vi "Controller Acquisition and Actuation Loop.vi"(4 "Iteration duration":u64, 5 "Missed iteration count":u32, 6 "Timestamp":u64, 7 "Sync Objects":T3, 8 "error in (no error)":errorcluster, 9 "PS Variables":T1, 10 "BPM Variables":T2, 11 "FOFB Configuration":T6={"FOFB Parameters"={"Network"={"FOFB Controller IP"="", "LNLS Control Network IP"="", "LNLS Control Network Power Supplies TCP Port"=0, "LNLS Control Network FOFB Configuration TCP Port"=0, "LNLS Control Network BPMs TCP Port"=0, "Monitoring Data TCP Port"=0, "Fast Archiver TCP Port"=0, "Fast Command TCP Port"=0, "TCP Listening Timeout"=0}, "Fast Acquisition"={"Sampling Period"=0, "Data Buffer Size"=0, "Monitoring Period"=0}, "Acquisition Network"=[], "Actuation Network"=[]}, "Number of Acquisition Chassis"=0, "Number of Actuation Chassis"=0, "Number of BPM Readings"=0, "BPM Reading Names"=[], "Selected BPM Readings"=[0, 1, 2, 3, 4, 5, 6, 7, 8, 9, 10, 11, 12, 13, 14, 15, 16, 17, 18, 19, 20, 21, 22, 23, 24, 25, 26, 27, 28, 29, 30, 31, 32, 33, 34, 35, 36, 37, 38, 39, 40, 41, 42, 43, 44, 45, 46, 47, 48, 49], "Number of Correctors"=0, "Corrector Names"=[], "Selected Correctors"=[0, 1, 2, 3, 4, 5, 6, 7, 8, 9, 10, 11, 12, 13, 14, 15, 16, 17, 18, 19, 20, 21, 22, 23, 24, 25, 26, 27, 28, 29, 30, 31, 32, 33, 34, 35, 36, 37, 38, 39, 40, 41, 42, 43, 44, 45, 46, 47, 48, 49], "Response Matrix"=[], "Reference Orbit"=[], "Correction Matrix"=[], "FPGA Filter Sets"=[], "Acquisition Chassis Names"=[], "Actuation Chassis Names"=[], "Acquisition Variables"=[], "Actuation Variables"=[], "PS Matrix Mapping"=[], "Inverse PS Matrix Mapping"=[], "BPM Matrix Mapping"=[], "Inverse BPM Matrix Mapping"=[], "BPM Planes"=[], "Corrector Planes"=[]}) -> (0 "error out":errorcluster)   [LabVIEW 2011, in "Controller VIs.lvlib"]
doc: "Continuously performs acquisition of all input variables (BPM readings, Power Supply readings, etc.) and forwards data to the <b>Decimated Acquisition Loop</b>."
uses:
  Controller VIs.lvlib
  Types Definitions/Type FOFB Configuration.ctl
  Types Definitions/Type FOFB Parameters.ctl
  Types Definitions/Type Network Configuration.ctl
  Types Definitions/Type FA Configuration.ctl
  Types Definitions/Type Acquisition Network Configuration.ctl
  Types Definitions/Type Actuation Network Configuration.ctl
  Types Definitions/Type Synchronization Objects.ctl
  Types Definitions/Type Blocking Synchronization Objects.ctl
  Types Definitions/Type Monitoring Data.ctl
  Types Definitions/Type Operation Mode State.ctl
  Types Definitions/Type Diagnostics Data.ctl
  Types Definitions/Type CPU Loads Array.ctl
  Types Definitions/Type CPU Loads.ctl
  Types Definitions/Type Non-blocking Synchronization Objects.ctl
  Types Definitions/Type FOFB Variables.ctl
  Types Definitions/Type Actuation State.ctl
  Types Definitions/Type BPM Variables.ctl
  Types Definitions/Type PS Variables.ctl
  Controller Write UINT8.vi
  Controller Write PS Setpoints.vi
  Controller Write Boolean.vi
  Controller Write FXP22.4.vi
  Controller Write UINT16.vi
  Controller Read FXP20.5.vi
  Controller Read UINT8.vi
  Controller Write FXP20.5.vi
  Type Definitions.lvlib
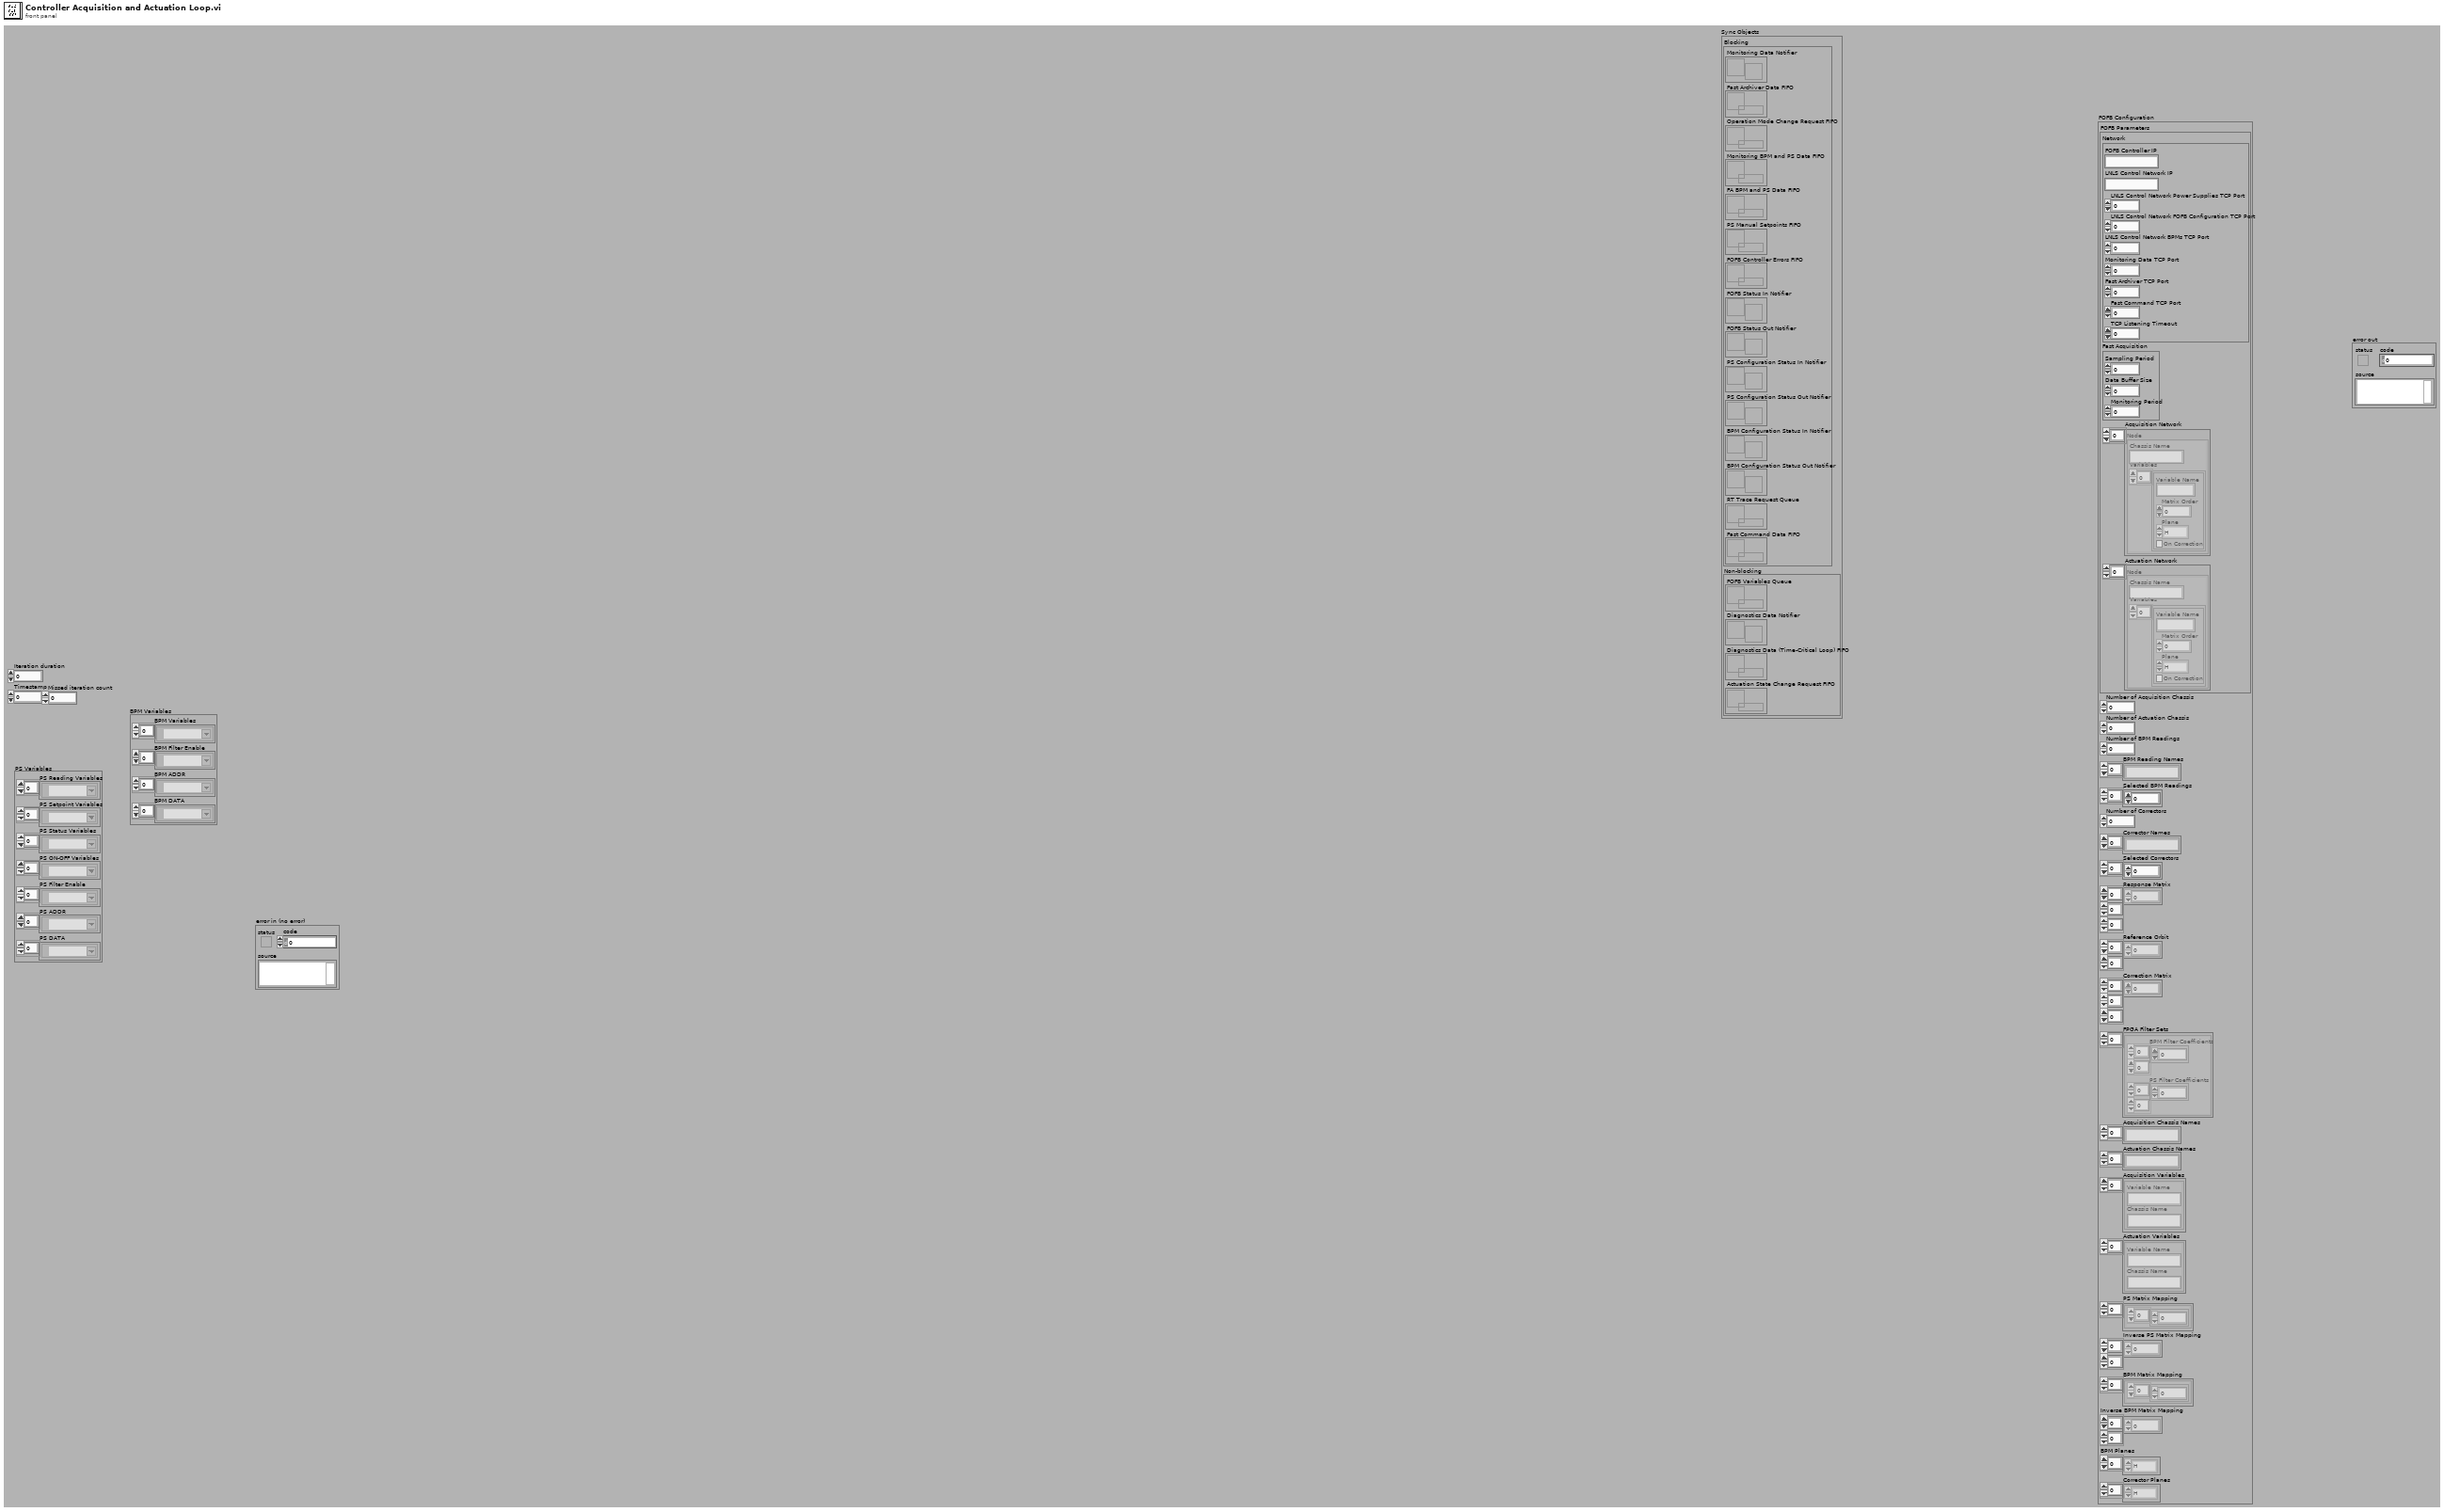
[diagram p1: front panel]
types:
  T1 = typedef "Type Definitions.lvlib/Type PS Variables.ctl" = cluster{"PS Reading Variables":refnum<k21>[], "PS Setpoint Variables":refnum<k21>[], "PS Status Variables":refnum<k21>[], "PS ON-OFF Variables":refnum<k21>[], "PS Filter Enable":refnum<k21>[], "PS ADDR":refnum<k21>[], "PS DATA":refnum<k21>[]}
  T2 = typedef "Type Definitions.lvlib/Type BPM Variables.ctl" = cluster{"BPM Variables":refnum<k21>[], "BPM Filter Enable":refnum<k21>[], "BPM ADDR":refnum<k21>[], "BPM DATA":refnum<k21>[]}
  T3 = typedef "Type Definitions.lvlib/Type Synchronization Objects.ctl" = cluster{"Blocking":T4, "Non-blocking":T5}
  T4 = typedef "Type Definitions.lvlib/Type Blocking Synchronization Objects.ctl" = cluster{"Monitoring Data Notifier":refnum<notifier>, "Fast Archiver Data FIFO":refnum<queue>, "Operation Mode Change Request FIFO":refnum<k33>, "Monitoring BPM and PS Data FIFO":refnum<k33>, "FA BPM and PS Data FIFO":refnum<k33>, "PS Manual Setpoints FIFO":refnum<k33>, "FOFB Controller Errors FIFO ":refnum<k33>, "FOFB Status In Notifier":refnum<notifier>, "FOFB Status Out Notifier":refnum<notifier>, "PS Configuration Status In Notifier":refnum<notifier>, "PS Configuration Status Out Notifier":refnum<notifier>, "BPM Configuration Status In Notifier":refnum<notifier>, "BPM Configuration Status Out Notifier":refnum<notifier>, "RT Trace Request Queue":refnum<queue>, "Fast Command Data FIFO":refnum<k33>}
  T5 = typedef "Type Definitions.lvlib/Type Non-blocking Synchronization Objects.ctl" = cluster{"FOFB Variables Queue":refnum<queue>, "Diagnostics Data Notifier":refnum<notifier>, "Diagnostics Data (Time-Critical Loop) FIFO":refnum<k33>, "Actuation State Change Request FIFO":refnum<k33>}
  T6 = typedef "Type Definitions.lvlib/Type FOFB Configuration.ctl" = cluster{"FOFB Parameters":T7, "Number of Acquisition Chassis":i32, "Number of Actuation Chassis":i32, "Number of BPM Readings":i32, "BPM Reading Names":string[], "Selected BPM Readings":u32[], "Number of Correctors":i32, "Corrector Names":string[], "Selected Correctors":u32[], "Response Matrix":dbl[][][], "Reference Orbit":dbl[][], "Correction Matrix":dbl[][][], "FPGA Filter Sets":cluster{"BPM Filter Coefficients":dbl[][], "PS Filter Coefficients":dbl[][]}[], "Acquisition Chassis Names":string[], "Actuation Chassis Names":string[], "Acquisition Variables":cluster{"Variable Name":string, "Chassis Name":string}[], "Actuation Variables":cluster{"Variable Name":string, "Chassis Name":string}[], "PS Matrix Mapping":cluster{u32[]}[], "Inverse PS Matrix Mapping":u32[][], "BPM Matrix Mapping":cluster{u32[]}[], "Inverse BPM Matrix Mapping":u32[][], "BPM Planes":enum8{"H", "V"}[], "Corrector Planes":enum8{"H", "V"}[]}
  T7 = typedef "Type Definitions.lvlib/Type FOFB Parameters.ctl" = cluster{"Network":T8, "Fast Acquisition":T9, "Acquisition Network":T10, "Actuation Network":T11}
  T8 = typedef "Type Definitions.lvlib/Type Network Configuration.ctl" = cluster{"FOFB Controller IP":string, "LNLS Control Network IP":string, "LNLS Control Network Power Supplies TCP Port":u16, "LNLS Control Network FOFB Configuration TCP Port":u16, "LNLS Control Network BPMs TCP Port":u16, "Monitoring Data TCP Port":u16, "Fast Archiver TCP Port":u16, "Fast Command TCP Port":u16, "TCP Listening Timeout":i32}
  T9 = typedef "Type Definitions.lvlib/Type FA Configuration.ctl" = cluster{"Sampling Period":u32, "Data Buffer Size":u32, "Monitoring Period":u32}
  T10 = typedef "Type Definitions.lvlib/Type Acquisition Network Configuration.ctl" = cluster{"Chassis Name":string, "Variables":cluster{"Variable Name":string, "Matrix Order":u32, "Plane":enum8{"H", "V"}, "On Correction":bool}[]}[]
  T11 = typedef "Type Definitions.lvlib/Type Actuation Network Configuration.ctl" = cluster{"Chassis Name":string, "Variables":cluster{"Variable Name":string, "Matrix Order":u32, "Plane":enum8{"H", "V"}, "On Correction":bool}[]}[]
  T12 = typedef "Type Definitions.lvlib/Type Actuation State.ctl" = enum8{"Only reading", "Manual", "FOFB Initialization", "FOFB", "FOFB Stopping"}
  T13 = typedef "Type Definitions.lvlib/Type FOFB Variables.ctl" = cluster{"Reference Orbit":dbl[], "Response Matrix":dbl[][], "Correction Matrix":dbl[][], "FPGA Filter":cluster{"BPM Filter Coefficients":dbl[][], "PS Filter Coefficients":dbl[][]}, "Selected BPM Readings":u32[], "Selected Correctors":u32[], "BPM Planes":enum8{"H", "V"}[], "Corrector Planes":enum8{"H", "V"}[], "Fast Command Enabled":bool, "Horizontal Gain":dbl, "Vertical Gain":dbl, "Horizontal Distortion Threshold":dbl, "Vertical Distortion Threshold":dbl}
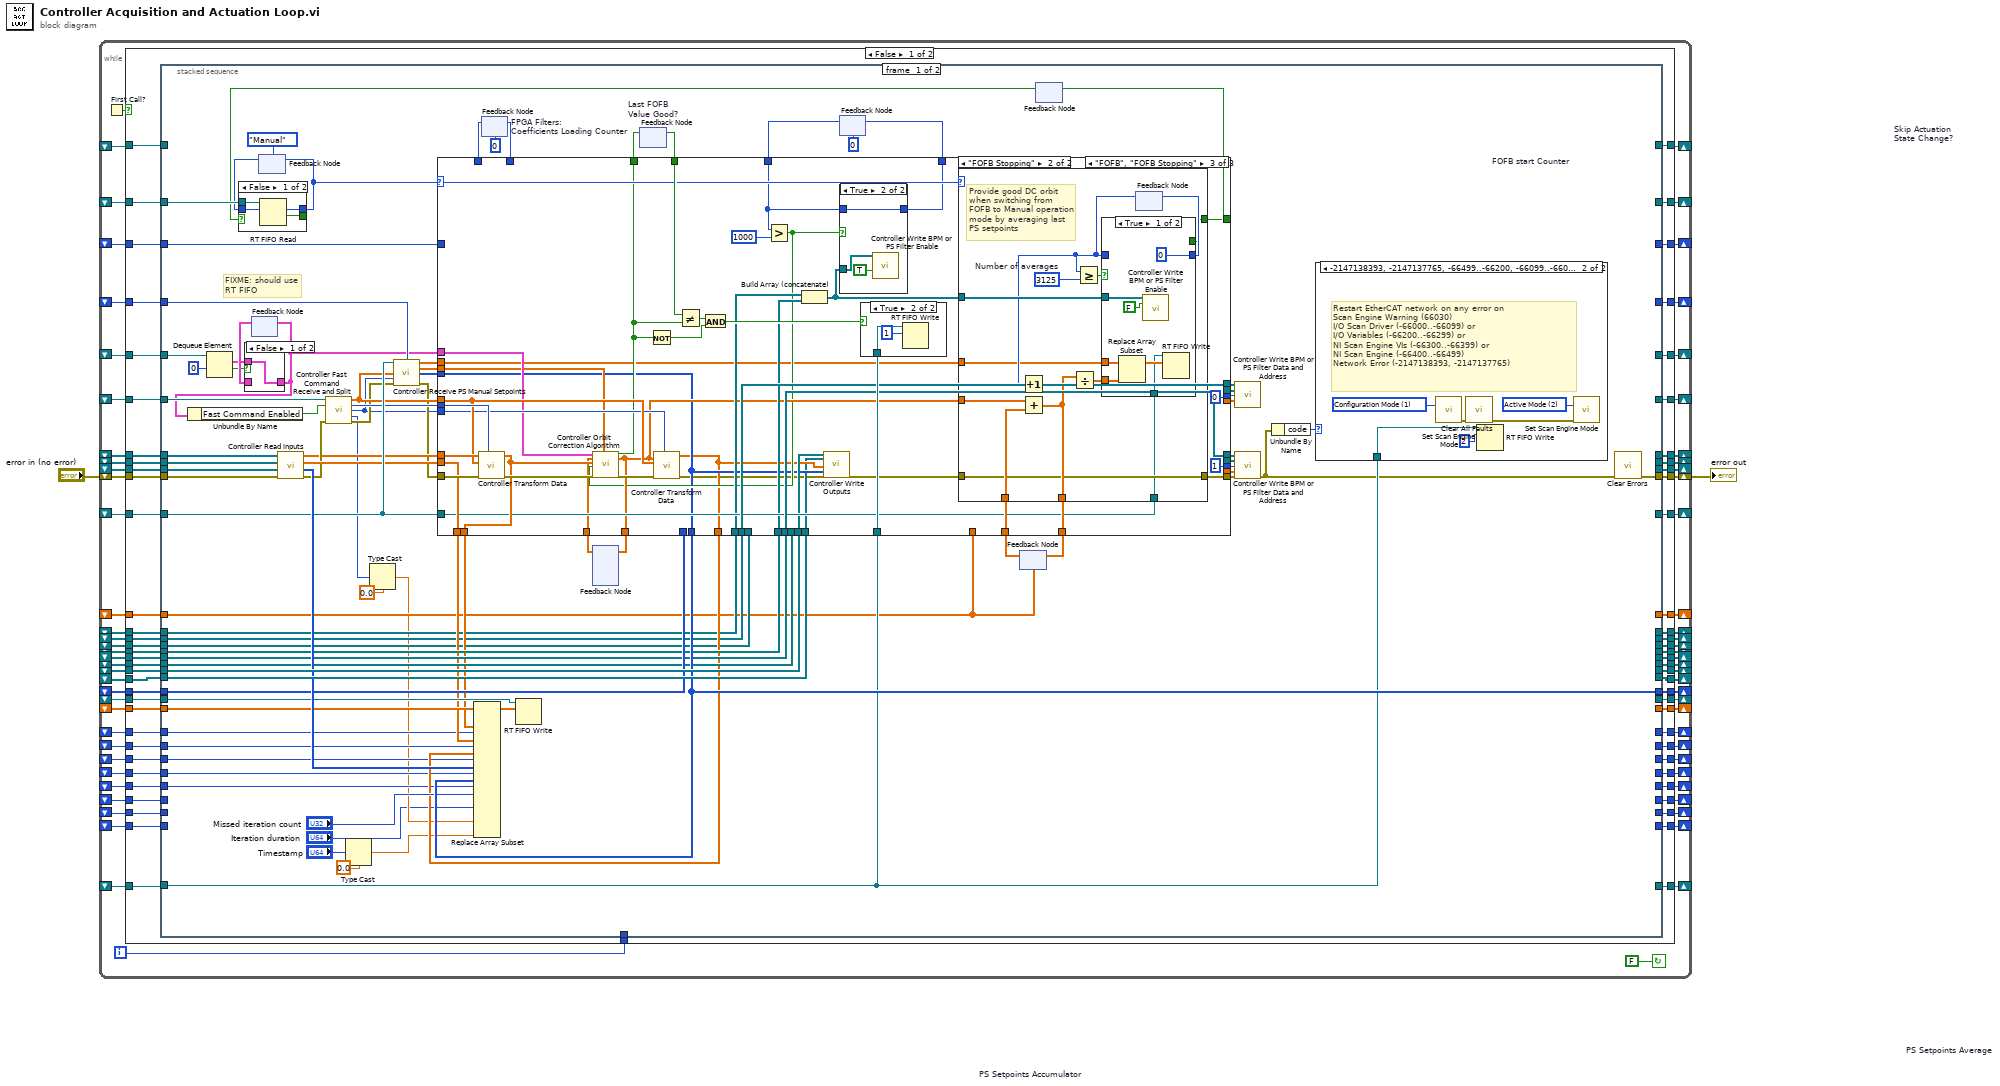
[diagram p0: block diagram]
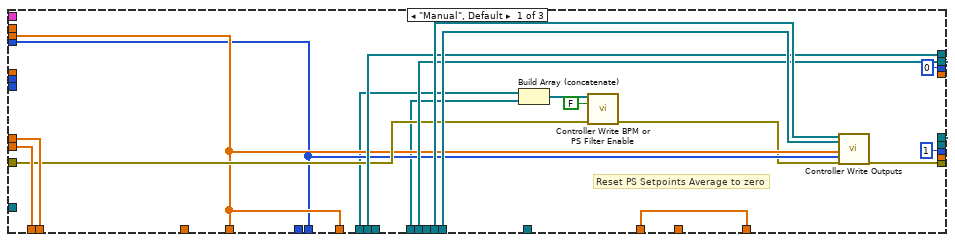
[diagram p4: hidden frame]
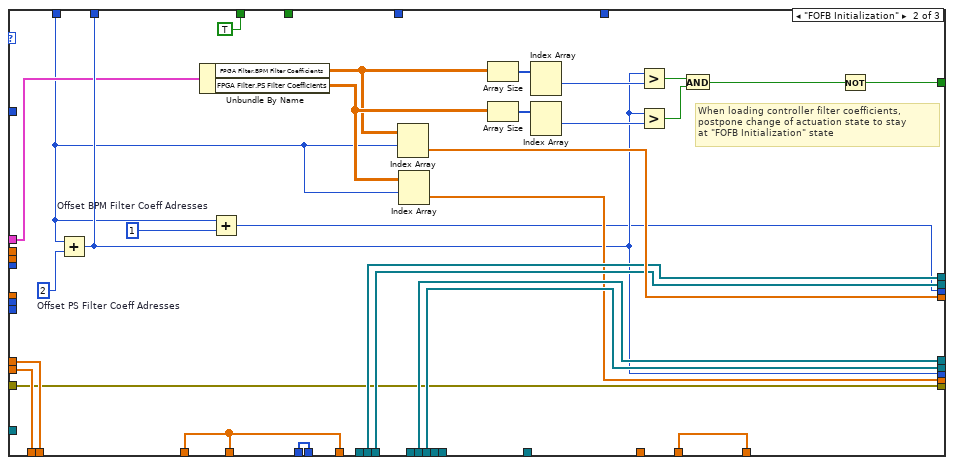
[diagram p5: hidden frame]
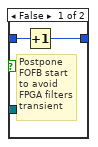
[diagram p6: hidden frame]
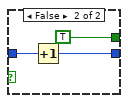
[diagram p8: hidden frame]
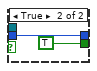
[diagram p10: hidden frame]
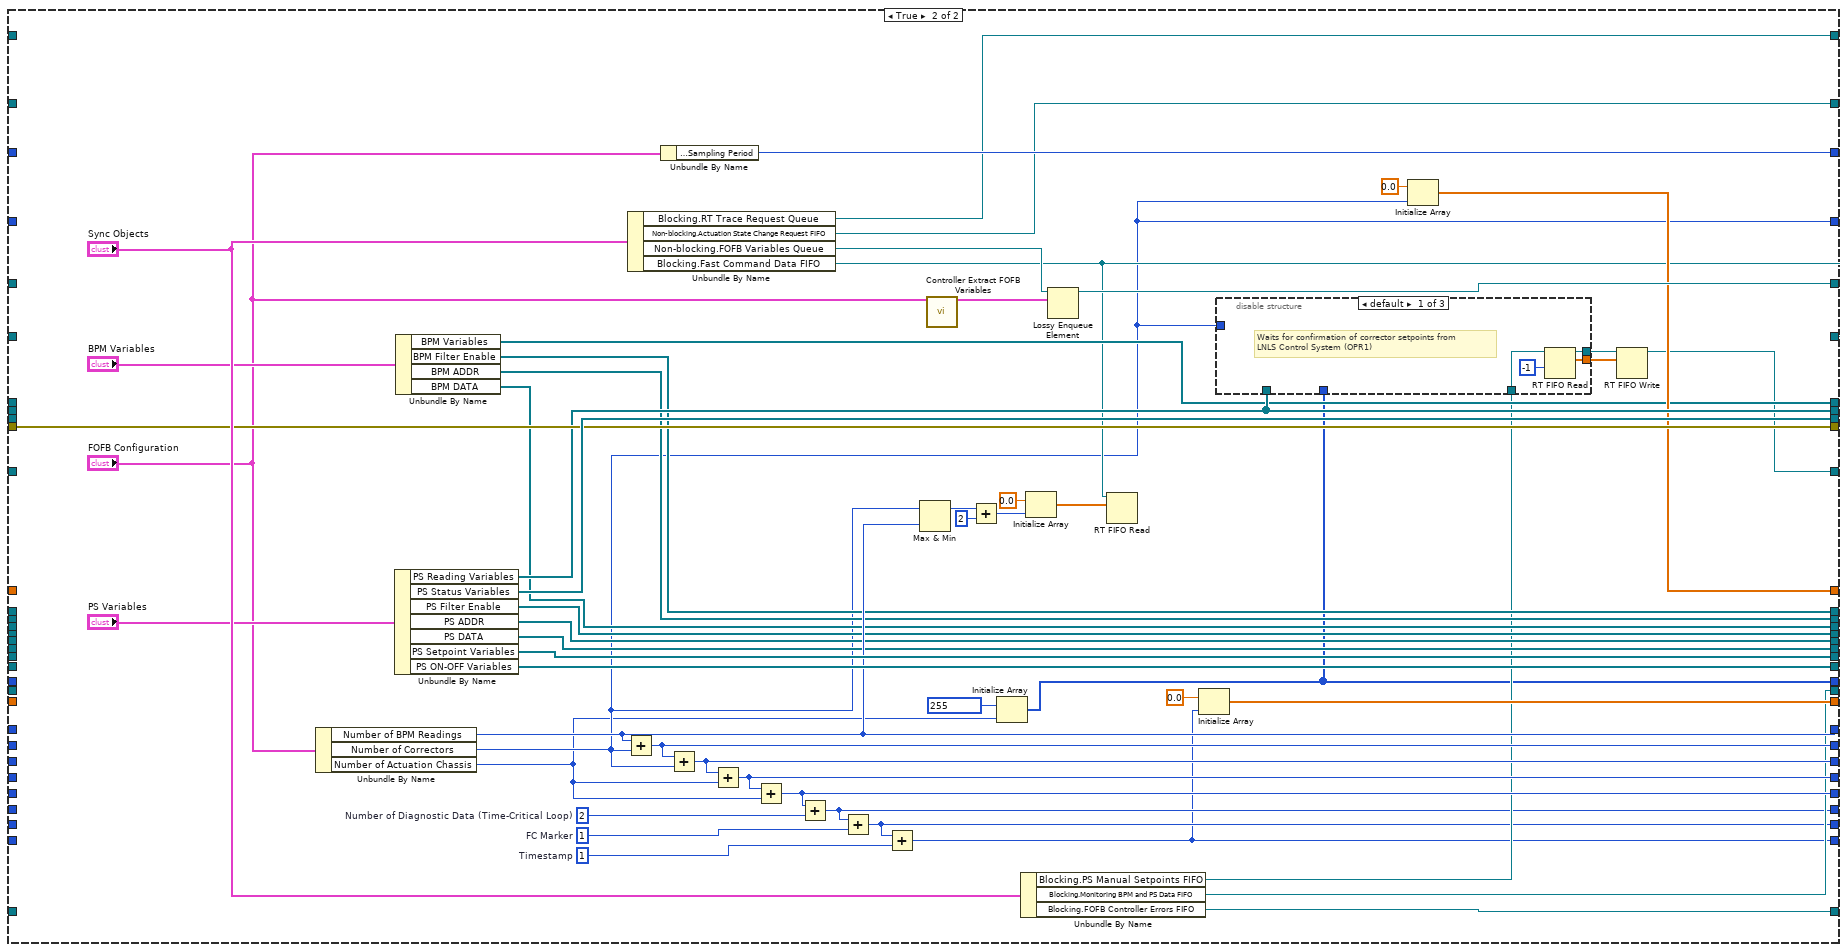
[diagram p12: hidden frame]
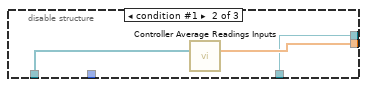
[diagram p13: hidden frame]
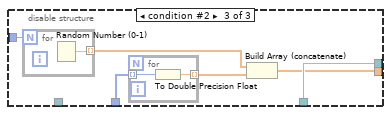
[diagram p14: hidden frame]
diagram:
  n1 = while {
    shift-right: [w56] -> w2
    shift-left: "error in (no error)" -> [w27]
    shift-right: [w52] -> _
    shift-left: _ -> [w64]
    shift-right: [w51] -> _
    shift-left: _ -> [w69]
    shift-right: [w50] -> _
    shift-left: _ -> [w68]
    shift-right: [w49] -> _
    shift-left: _ -> [w66]
    shift-right: [w10] -> _
    shift-left: _ -> [w55]
    shift-right: [w48] -> _
    shift-left: _ -> [w65]
    shift-right: [w47] -> _
    shift-left: _ -> [w63]
    shift-right: [w46] -> _
    shift-left: _ -> [w67]
    shift-right: [w45] -> _
    shift-left: _ -> [w60]
    shift-right: [w44] -> _
    shift-left: _ -> [w62]
    shift-right: [w43] -> _
    shift-left: _ -> [w59]
    shift-right: [w42] -> _
    shift-left: _ -> [w61]
    shift-right: [w41] -> _
    shift-left: _ -> [w58]
    shift-right: [w40] -> _
    shift-left: _ -> [w57]
    shift-right: [w39] -> _
    shift-left: _ -> [w36]
    shift-right: [w38] -> _
    shift-left: _ -> [w35]
    shift-right: [w37] -> _
    shift-left: _ -> [w34]
    shift-right: [w32] -> _
    shift-left: _ -> [w33]
    shift-right: [w31] -> _
    shift-left: _ -> [w30]
    shift-right: [w29] -> _
    shift-left: _ -> [w28]
    shift-right: [w25] -> _
    shift-left: _ -> [w26]
    shift-right: [w23] -> _
    shift-left: _ -> [w24]
    shift-right: [w21] -> _
    shift-left: _ -> [w20]
    shift-right: [w22] -> _
    shift-left: _ -> [w19]
    shift-right: [w18] -> _
    shift-left: _ -> [w17]
    shift-right: [w16] -> _
    shift-left: _ -> [w13]
    shift-right: [w14] -> _
    shift-left: _ -> [w11]
    shift-right: [w15] -> _
    shift-left: _ -> [w12]
    shift-right: [w9] -> _
    shift-left: _ -> [w7]
    shift-right: [w8] -> _
    shift-left: _ -> [w6]
    shift-right: [w5] -> _
    shift-left: _ -> [w4]
    i -> [w3]
    stop <- FALSE continue-if-true
    n2 = First Call?() -> (First Call?: T/F=w53:bool)
    n3 = case shown="False" w53 {
      tunnel: w69 -> [w134 _]
      tunnel: w68 -> [w133 _]
      tunnel: w67 -> [w132 _]
      tunnel: w66 -> [w131 _]
      tunnel: w65 -> [w130 _]
      tunnel: w64 -> [w129 _]
      tunnel: w63 -> [w128 _]
      tunnel: w62 -> [w127 _]
      tunnel: w61 -> [w126 _]
      tunnel: w60 -> [w125 _]
      tunnel: w59 -> [w124 _]
      tunnel: w58 -> [w123 _]
      tunnel: w57 -> [w122 _]
      tunnel: [w121 w428] -> w56
      tunnel: w27 -> [w120 w428]
      tunnel: w55 -> [w119 _]
      tunnel: [w117 w403] -> w52
      tunnel: [w116 w414] -> w51
      tunnel: [w115 w427] -> w50
      tunnel: [w114 w441] -> w49
      tunnel: [w113 w440] -> w48
      tunnel: [w112 w419] -> w47
      tunnel: [w111 w439] -> w46
      tunnel: [w110 w438] -> w45
      tunnel: [w109 w422] -> w44
      tunnel: [w108 w437] -> w43
      tunnel: [w107 w436] -> w42
      tunnel: [w106 w435] -> w41
      tunnel: [w105 w424] -> w40
      tunnel: [w100 w404] -> w39
      tunnel: [w99 w405] -> w38
      tunnel: [w98 w429] -> w37
      tunnel: w36 -> [w102 _]
      tunnel: w35 -> [w101 _]
      tunnel: w34 -> [w118 _]
      tunnel: w33 -> [w104 _]
      tunnel: [w103 w402] -> w32
      tunnel: w30 -> [w97 _]
      tunnel: [w96 w398] -> w31
      tunnel: [w94 w425] -> w29
      tunnel: w28 -> [w95 _]
      tunnel: w26 -> [w93 _]
      tunnel: [w92 w410] -> w25
      tunnel: w24 -> [w91 _]
      tunnel: [w90 w420] -> w23
      tunnel: [w87 w418] -> w22
      tunnel: [w86 w417] -> w21
      tunnel: w20 -> [w89 _]
      tunnel: w19 -> [w88 _]
      tunnel: [w84 w415] -> w18
      tunnel: w17 -> [w85 _]
      tunnel: [w80 w413] -> w16
      tunnel: [w79 w412] -> w15
      tunnel: [w78 w411] -> w14
      tunnel: w13 -> [w83 _]
      tunnel: w12 -> [w82 _]
      tunnel: w11 -> [w81 _]
      tunnel: [w77 w401] -> w10
      tunnel: [w73 w395] -> w9
      tunnel: [w74 w394] -> w8
      tunnel: w7 -> [w76 _]
      tunnel: w6 -> [w75 _]
      tunnel: [w72 w390] -> w5
      tunnel: w4 -> [w71 _]
      tunnel: w3 -> [w70 _]
      frame False {
        n4 = stacked-sequence {
          tunnel: w134 -> [w222 w388]
          tunnel: w133 -> [w221 w387]
          tunnel: w132 -> [w220 w382]
          tunnel: w131 -> [w219 w386]
          tunnel: w130 -> [w218 w384]
          tunnel: w129 -> [w217 w389]
          tunnel: w128 -> [w201 w383]
          tunnel: w127 -> [w142 w380]
          tunnel: w126 -> [w144 w378]
          tunnel: w125 -> [w215 w381]
          tunnel: w124 -> [w143 w379]
          tunnel: w123 -> [w141 w377]
          tunnel: w122 -> [w140 w376]
          tunnel: [w208 _] -> w121
          tunnel: w120 -> [w194 _]
          tunnel: w119 -> [w193 w385]
          tunnel: w102 -> [w214 w375]
          tunnel: w118 -> [w210 w373]
          tunnel: w101 -> [w192 w374]
          tunnel: [_ w389] -> w117
          tunnel: [_ w388] -> w116
          tunnel: [_ w387] -> w115
          tunnel: [_ w386] -> w114
          tunnel: [_ w385] -> w77
          tunnel: [_ w384] -> w113
          tunnel: [_ w383] -> w112
          tunnel: [_ w382] -> w111
          tunnel: [_ w381] -> w110
          tunnel: [_ w380] -> w109
          tunnel: [_ w379] -> w108
          tunnel: [_ w378] -> w107
          tunnel: [_ w377] -> w106
          tunnel: [_ w376] -> w105
          tunnel: [_ w375] -> w100
          tunnel: [_ w374] -> w99
          tunnel: [_ w373] -> w98
          tunnel: w104 -> [w213 _]
          tunnel: [w212 _] -> w103
          tunnel: w97 -> [_ w372]
          tunnel: [_ w372] -> w96
          tunnel: w95 -> [w211 w371]
          tunnel: [_ w371] -> w94
          tunnel: w93 -> [w205 w370]
          tunnel: [_ w370] -> w92
          tunnel: w91 -> [w204 w369]
          tunnel: [_ w369] -> w90
          tunnel: w89 -> [w203 w367]
          tunnel: w88 -> [w202 w368]
          tunnel: [_ w368] -> w87
          tunnel: [_ w367] -> w86
          tunnel: w85 -> [w191 w366]
          tunnel: [_ w366] -> w84
          tunnel: w83 -> [w197 w365]
          tunnel: w82 -> [w196 w364]
          tunnel: w81 -> [w195 w363]
          tunnel: [_ w365] -> w80
          tunnel: [_ w364] -> w79
          tunnel: [_ w363] -> w78
          tunnel: w76 -> [_ w361]
          tunnel: w75 -> [_ w362]
          tunnel: [_ w362] -> w74
          tunnel: [_ w361] -> w73
          tunnel: [_ w360] -> w72
          tunnel: w71 -> [_ w360]
          tunnel: w70 -> [_ _]
          frame #0 {
            # "FIXME: should use\nRT FIFO"
            n5 = Dequeue Element(queue=w211, timeout in ms (-1)=0) -> (element=w146:T13, timed out?=w147:bool)  [unwired: 1 in, 2 out]
            n6 = feedback #1() -> (w148:T13)  [unwired: 1 in]
            n7 = case shown="False" w147 {
              tunnel: [w223 w224] -> w151
              tunnel: w146 -> [w223 _]
              tunnel: w148 -> [_ w224]
              frame False {
              }
              frame True {
              }
            }
            n8 = Unbundle By Name(w151) -> ("Fast Command Enabled"=w186:bool)
            n9 = feedback-in #1(w151) -> ()
            n10 = feedback #2(Type_Actuation_State."Manual" ("Actuation State")) -> (w184:T12)
            n11 = call "Controller Read Inputs.vi"("error in (no error)"=w194, "PS Status Variables"=w219, "PS Reading Variables"=w221, "BPM Variables"=w222) -> ("error out"=w189:errorcluster, "PS Status (per PS Rack)"=w216:u8[], "PS Readings"=w190:dbl[], "BPM Readings"=w188:dbl[])  [unwired: 4 in]
            n12 = call "Controller Fast Command Receive and Split.vi"("Fast Command FIFO"=w205, "Fast Command Enabled"=w186, "error in (no error)"=w189) -> ("FC Data"=w182:sgl[], "FC BPM Mode"=w183:u16, "FC PS Mode"=w179:u16, "FC Marker"=w137:u32, "error out"=w181:errorcluster)  [unwired: 8 in]
            n13 = Type Cast(type=0.0 ("double precision float"), x="Timestamp") -> (*(type *) &x=w139:dbl)
            n14 = Type Cast(type=0.0 ("double precision float"), x=w137) -> (*(type *) &x=w136:dbl)
            n15 = call "Controller Receive PS Manual Setpoints.vi"("PS Setpoints FIFO"=w192, "Number of Correctors"=w193, "FC PS Setpoints"=w182, "FC PS Mode"=w179, "error in (no error)"=w181) -> ("Raw PS Setpoints + PS ON-OFF"=w176:dbl[], "PS Setpoints"=w177:dbl[], "PS ON-OFF (per PS Rack)"=w178:u8[], "error out"=w180:errorcluster)  [unwired: 6 in, 1 out]
            n16 = feedback #3 "FPGA Filters:\nCoefficients Loading Counter"(u16 0 ("Base address")) -> (w154:u16)
            n17 = feedback #4 "PS Setpoints Accumulator"() -> (w174:dbl[])  [unwired: 1 in]
            n18 = feedback #5 "Last FOFB\nValue Good?"() -> (w167:bool)  [unwired: 1 in]
            n19 = feedback #6 "FOFB start Counter"(0) -> (w158:i32)
            n20 = feedback #7 "PS Setpoints Average"(w191) -> (w165:dbl[])
            n21 = feedback #8 "Skip Actuation\nState Change?"() -> (w150:bool)  [unwired: 1 in]
            n22 = case shown="False" w150 {
              tunnel: w217 -> [w357 _]
              tunnel: w184 -> [w356 w359]
              tunnel: [w355 w359] -> w175
              tunnel: [w354 TRUE ("empty?")] -> _
              frame False {
                n23 = RT FIFO Read(0:w357, 1:w356) -> (9:w355:T12, 10:w354:bool)  [unwired: 2 in, 3 out]
              }
              frame True {
              }
            }
            n24 = feedback-in #2(w175) -> ()
            n25 = case shown="\"FOFB\", \"FOFB Stopping\"" w175 {
              selector: w175 -> [_ _ w307]
              tunnel: [w246 w254 w306] -> w172
              tunnel: w180 -> [w239 w254 w320]
              tunnel: w188 -> [w243 w275 w319]
              tunnel: w218 -> [w248 _ w285]
              tunnel: w220 -> [w247 _ w282]
              tunnel: w174 -> [_ w273 w287]
              tunnel: [w237 w253 w284] -> w212
              tunnel: w213 -> [_ w253 _]
              tunnel: w151 -> [_ w255 w311]
              tunnel: w210 -> [_ _ w310]
              tunnel: w182 -> [_ _ w317]
              tunnel: w183 -> [_ _ w318]
              tunnel: w179 -> [_ _ w316]
              tunnel: [_ w277 w305] -> w152
              tunnel: w190 -> [w242 w274 w301]
              tunnel: w204 -> [_ _ _]
              tunnel: w203 -> [w235 _ w294]
              tunnel: w202 -> [w245 w276 w297]
              tunnel: w201 -> [_ w272 _]
              tunnel: [_ w268 _] -> w171
              tunnel: [u16 1 w258 u16 1] -> w170
              tunnel: [_ w272 _] -> w163
              tunnel: [w245 w276 w297] -> w169
              tunnel: [_ TRUE w300] -> w168
              tunnel: w167 -> [_ _ w309]
              tunnel: [w244 w257 w304] -> w166
              tunnel: w165 -> [_ w257 w303]
              tunnel: w191 -> [w244 _ _]
              tunnel: [w243 w275 w302] -> w200
              tunnel: [w242 w274 w301] -> w199
              tunnel: [w238 w273 w292] -> w164
              tunnel: [w238 w273 w283] -> w198
              tunnel: w197 -> [_ w269 _]
              tunnel: w196 -> [w241 w270 w299]
              tunnel: w195 -> [w236 _ w295]
              tunnel: [_ w271 _] -> w162
              tunnel: [u16 0 w249 u16 0] -> w161
              tunnel: [w241 w270 w299] -> w160
              tunnel: [_ w269 _] -> w159
              tunnel: w158 -> [_ _ w290]
              tunnel: [_ _ w289] -> w157
              tunnel: [_ w258 _] -> w155
              tunnel: w154 -> [_ w251 _]
              tunnel: w178 -> [w237 _ w284]
              tunnel: w177 -> [w238 _ w286]
              tunnel: w192 -> [_ _ w296]
              tunnel: w176 -> [_ _ w288]
              frame "Manual", Default {
                # "Reset PS Setpoints Average to zero"
                n26 = Build Array (concatenate)(w236, w235) -> (w234:refnum<k21>[])
                n27 = call "Controller Write BPM or PS Filter Enable.vi"("BPM-PS Filter Enable"=w234, "Filter Enable"=FALSE, "error in"=w239) -> ("error out"=w233:errorcluster)  [unwired: 12 in]
                n28 = call "Controller Write Outputs.vi"("PS Setpoint Variables"=w248, "PS ON-OFF Variables"=w247, "PS Setpoints"=w238, "PS ON-OFF (per PS Rack)"=w237, "error in (no error)"=w233) -> ("error out"=w246:errorcluster)  [unwired: 14 in]
              }
              frame "FOFB Initialization" {
                w250 = u16 1  # Offset BPM Filter Coeff Adresses
                w252 = u16 2  # Offset PS Filter Coeff Adresses
                # "When loading controller filter coefficients,\npostpone change of actuation state to stay\nat \"FOFB Initialization\" state"
                n29 = Add(x=w251, y=w252) -> (x+y=w258:u16)
                n30 = Unbundle By Name(w255) -> ("FPGA Filter.BPM Filter Coefficients"=w259:dbl[][], "FPGA Filter.PS Filter Coefficients"=w264:dbl[][])
                n31 = Add(x=w251, y=w250) -> (x+y=w249:u16)
                n32 = Index Array(array=w259, index (row)=w251) -> (element=w271:dbl[])  [unwired: 1 in]
                n33 = Index Array(array=w264, index (row)=w251) -> (element=w268:dbl[])  [unwired: 1 in]
                n34 = Array Size(array=w259) -> (size(s)=w266:i32[])
                n35 = Array Size(array=w264) -> (size(s)=w265:i32[])
                n36 = Index Array(array=w266) -> (element #1=w261:i32)  [unwired: 2 in, 1 out]
                n37 = Index Array(array=w265) -> (element #1=w260:i32)  [unwired: 2 in, 1 out]
                n38 = Greater?(x=w258, y=w261) -> (0:w262:bool)
                n39 = Greater?(x=w258, y=w260) -> (0:w263:bool)
                n40 = And(x=w262, y=w263) -> (x .and. y?=w267:bool)
                n41 = Not(x=w267) -> (.not. x?=w277:bool)
              }
              frame "FOFB", "FOFB Stopping" {
                n42 = call "Controller Transform Data.vi"("Mode (Transparent)"=w318, "error in (no error)"=w320, "New Data"=w317, "Data"=w319) -> ("error out"=w313:errorcluster, "Transformed Data"=w302:dbl[])  [unwired: 6 in]
                n43 = Greater?(x=w290, y=1000) -> (0:w291:bool)
                n44 = call "Controller Orbit Correction Algorithm.vi"("FOFB Variables"=w311, "Corrector Kick Vector in"=w287, "Beam Position Vector"=w302, "Active?"=w291, "error in (no error)"=w313, "Corrector Kick Vector Manual Setpoint in"=w286) -> ("Good value?"=w300:bool, "Corrector Kick Vector out"=w292:dbl[], "error out"=w312:errorcluster)  [unwired: 11 in]
                n45 = Not(x=w300) -> (.not. x?=w314:bool)
                n46 = call "Controller Transform Data.vi"("Mode (Transparent)"=w316, "error in (no error)"=w312, "New Data"=w317, "Data"=w292) -> ("error out"=w281:errorcluster, "Transformed Data"=w283:dbl[])  [unwired: 6 in]
                n47 = Not Equal?(x=w309, y=w300) -> (x != y?=w308:bool)
                n48 = And(x=w308, y=w314) -> (x .and. y?=w315:bool)
                n49 = Build Array (concatenate)(w295, w294) -> (w293:refnum<k21>[])
                n50 = call "Controller Write Outputs.vi"("PS Setpoint Variables"=w285, "PS ON-OFF Variables"=w282, "PS Setpoints"=w283, "PS ON-OFF (per PS Rack)"=w284, "error in (no error)"=w281) -> ("error out"=w280:errorcluster)  [unwired: 14 in]
                n51 = case shown="True" w291 {
                  tunnel: w293 -> [_ w324]
                  tunnel: w290 -> [w322 w323]
                  tunnel: [w321 w323] -> w289
                  frame False {
                    # "Postpone \nFOFB start\nto avoid \nFPGA filters\ntransient"
                    n52 = Increment(x=w322) -> (x+1=w321:i32)
                  }
                  frame True {
                    n53 = call "Controller Write BPM or PS Filter Enable.vi"("BPM-PS Filter Enable"=w324, "Filter Enable"=TRUE) -> ()  [unwired: 13 in, 1 out]
                  }
                }
                n54 = case shown="True" w315 {
                  tunnel: w310 -> [_ w352]
                  frame False {
                  }
                  frame True {
                    n55 = RT FIFO Write(0:w352, 1:u16 1 ("element")) -> ()  [unwired: 3 in, 4 out]
                  }
                }
                n56 = case shown="\"FOFB Stopping\"" w307 {
                  tunnel: w280 -> [w327 w335]
                  tunnel: [w327 w335] -> w306
                  tunnel: [_ w334] -> w305
                  tunnel: w293 -> [_ w340]
                  tunnel: [w326 w336] -> w304
                  tunnel: w303 -> [w326 w337]
                  tunnel: w296 -> [_ w331]
                  tunnel: w292 -> [_ w330]
                  tunnel: w288 -> [_ w328]
                  frame "FOFB", Default {
                  }
                  frame "FOFB Stopping" {
                    w338 = 3125  # Number of averages
                    # "Provide good DC orbit\nwhen switching from\nFOFB to Manual operation\nmode by averaging last\nPS setpoints"
                    n57 = Add(x=w330, y=w337) -> (x+y=w336:dbl[])
                    n58 = feedback #9() -> (w329:i32)  [unwired: 1 in]
                    n59 = Increment(x=w329) -> (x+1=w333:i32)
                    n60 = Divide(x=w336, y=w333) -> (x/y=w332:dbl[])
                    n61 = Greater Or Equal?(x=w329, y=w338) -> (x >= y?=w339:bool)
                    n62 = case shown="True" w339 {
                      tunnel: [_ TRUE] -> w334
                      tunnel: [0 w351] -> w341
                      tunnel: w340 -> [w346 _]
                      tunnel: w329 -> [_ w349]
                      tunnel: w328 -> [w344 _]
                      tunnel: w332 -> [w343 _]
                      tunnel: w331 -> [w342 _]
                      frame True {
                        n63 = Replace Array Subset(array=w344, new element=w343) -> (w345:dbl[])  [unwired: 1 in]
                        n64 = call "Controller Write BPM or PS Filter Enable.vi"("BPM-PS Filter Enable"=w346, "Filter Enable"=FALSE) -> ()  [unwired: 13 in, 1 out]
                        n65 = RT FIFO Write(0:w342, 1:w345) -> ()  [unwired: 3 in, 4 out]
                      }
                      frame False {
                        n66 = Increment(x=w349) -> (x+1=w351:i32)
                      }
                    }
                    n67 = feedback-in #9(w341) -> ()
                  }
                }
              }
            }
            n68 = Replace Array Subset(array=w215, new element #1=w200, new element #2=w199, index #2=w142, new element #3=w198, index #3=w143, new element #4=w216, index #4=w144, new element #5=w212, index #5=w141, new element #6="Missed iteration count", index #6=w140, new element #7="Iteration duration", new element #8=w136, new element #9=w139) -> (w145:dbl[])  [unwired: 4 in]
            n69 = feedback-in #3(w155) -> ()
            n70 = RT FIFO Write(0:w214, 1:w145) -> ()  [unwired: 3 in, 4 out]
            n71 = feedback-in #4(w164) -> ()
            n72 = feedback-in #5(w168) -> ()
            n73 = feedback-in #6(w157) -> ()
            n74 = feedback-in #7(w166) -> ()
            n75 = feedback-in #8(w152) -> ()
            n76 = call "Controller Write BPM or PS Filter Data and Address.vi"("BPM-PS ADDR"=w160, "BPM-PS DATA"=w159, "Address"=w161, "Data"=w162) -> ()  [unwired: 11 in, 1 out]
            n77 = call "Controller Write BPM or PS Filter Data and Address.vi"("BPM-PS ADDR"=w169, "BPM-PS DATA"=w163, "Address"=w170, "Data"=w171, "error in"=w172) -> ("error out"=w185:errorcluster)  [unwired: 10 in]
            n78 = Unbundle By Name(w185) -> ("code"=w173:i32)
            n79 = case shown="-2147138393, -2147137765, -66499..-66200, -66099..-66000, 66030" w173 {
              tunnel: w210 -> [_ w226]
              frame 0, Default {
              }
              frame -2147138393, -2147137765, -66499..-66200, -66099..-66000, 66030 {
                w228 = 2 items=["Configuration Mode"=1, "Active Mode"=2] ("mode (Active Mode)")
                w229 = 1 items=["Configuration Mode"=1, "Active Mode"=2] ("mode (Active Mode)")
                # "Restart EtherCAT network on any error on \nScan Engine Warning (66030)\nI/O Scan Driver\t(-66000..-66099) or\nI/O Variables\t(-66200..-66299) or\nNI Scan Engine VIs\t(-66300..-66399) or\nNI Scan Engine (-66400..-66499)\nNetwork Error (-2147138393, -2147137765)"
                n80 = call <vilib>:"Set Scan Engine Mode.vi"("mode (Active Mode)"=w229) -> ("error out"=w230:errorcluster)  [unwired: 14 in]
                n81 = call <vilib>:"Clear All Faults.vi"("error in (no error)"=w230) -> ("error out"=w227:errorcluster)  [unwired: 1 in, 9 out]
                n82 = RT FIFO Write(0:w226, 1:u16 2 ("element")) -> ()  [unwired: 3 in, 4 out]
                n83 = call <vilib>:"Set Scan Engine Mode.vi"("mode (Active Mode)"=w228, "error in (no error)"=w227) -> ()  [unwired: 13 in, 1 out]
              }
            }
            n84 = call <vilib>:"Clear Errors.vi"("error in (no error)"=w185) -> ("error out"=w208:errorcluster)  [unwired: 6 in]
          }
          frame #1 {
          }
        }
      }
      frame True {
        w397 = 1  # FC Marker
        w396 = 1  # Timestamp
        w399 = 2  # Number of Diagnostic Data (Time-Critical Loop)
        n85 = Unbundle By Name("FOFB Configuration") -> ("Number of BPM Readings"=w422:i32, "Number of Correctors"=w401:i32, "Number of Actuation Chassis"=w400:i32)
        n86 = Unbundle By Name("PS Variables") -> ("PS Reading Variables"=w427:refnum<k21>[], "PS Status Variables"=w441:refnum<k21>[], "PS Filter Enable"=w417:refnum<k21>[], "PS ADDR"=w418:refnum<k21>[], "PS DATA"=w419:refnum<k21>[], "PS Setpoint Variables"=w440:refnum<k21>[], "PS ON-OFF Variables"=w439:refnum<k21>[])
        n87 = Unbundle By Name("BPM Variables") -> ("BPM Variables"=w414:refnum<k21>[], "BPM Filter Enable"=w411:refnum<k21>[], "BPM ADDR"=w412:refnum<k21>[], "BPM DATA"=w413:refnum<k21>[])
        n88 = Add(x=w422, y=w401) -> (x+y=w437:i32)
        n89 = Unbundle By Name("Sync Objects") -> ("Blocking.RT Trace Request Queue"=w390:refnum<queue>, "Non-blocking.Actuation State Change Request FIFO"=w403:refnum<k33>, "Non-blocking.FOFB Variables Queue"=w425:refnum<queue>, "Blocking.Fast Command Data FIFO"=w410:refnum<k33>)
        n90 = Unbundle By Name("FOFB Configuration") -> ("FOFB Parameters.Fast Acquisition.Sampling Period"=w420:u32)
        n91 = Add(x=w437, y=w401) -> (x+y=w436:i32)
        n92 = Add(x=w436, y=w400) -> (x+y=w435:i32)
        n93 = Add(x=w435, y=w400) -> (x+y=w424:i32)
        n94 = Add(x=w424, y=w399) -> (x+y=w398:i32)
        n95 = Add(x=w398, y=w397) -> (x+y=w395:i32)
        n96 = Add(x=w395, y=w396) -> (x+y=w394:i32)
        n97 = Max & Min(x=w401, y=w422) -> (max(x,y)=w393:i32)  [unwired: 1 out]
        n98 = call "Controller Extract FOFB Variables.vi"("FOFB Configuration"="FOFB Configuration") -> ("FOFB Variables"=w426:T13)  [unwired: 13 in, 1 out]
        n99 = Add(x=w393, y=2) -> (x+y=w392:i32)
        n100 = Initialize Array(u8 255, w400) -> (w402:u8[])
        n101 = Unbundle By Name("Sync Objects") -> ("Blocking.PS Manual Setpoints FIFO"=w406:refnum<k33>, "Blocking.Monitoring BPM and PS Data FIFO"=w404:refnum<k33>, "Blocking.FOFB Controller Errors FIFO"=w429:refnum<k33>)
        n102 = Initialize Array(sgl 0.0, w392) -> (w409:sgl[])
        n103 = Lossy Enqueue Element(queue=w425, element=w426) -> ()  [unwired: 1 in, 4 out]
        n104 = RT FIFO Read(0:w410, 1:w409) -> ()  [unwired: 2 in, 5 out]
        n105 = Initialize Array(0.0 ("element"), w394) -> (w438:dbl[])
        n106 = disable-structure shown="default" {
          disable-tunnel: [w442 w448 w449] -> w407
          disable-tunnel: w406 -> [w445 w446 w454]
          disable-tunnel: w427 -> [_ w447 _]
          disable-tunnel: [w443 w446 w454] -> w408
          disable-tunnel: w401 -> [_ _ w453]
          disable-tunnel: w402 -> [_ _ w452]
          frame condition #0 (active) {
            # "Waits for confirmation of corrector setpoints from\nLNLS Control System (OPR1)"
            n107 = RT FIFO Read(0:w445, 2:-1 ("timeout in ms (0)")) -> (8:w443:refnum<k33>, 9:w442:dbl[])  [unwired: 2 in, 3 out]
          }
          frame condition #1 {
            n108 = call "Controller Average Readings Inputs.vi"("PS Reading Variables"=w447) -> ("PS"=w448:dbl[])  [unwired: 11 in, 3 out]
          }
          frame condition #2 {
            n109 = for {
              N: w453 -> [_]
              tunnel: [w457] -> w450 mode=indexing
              n110 = Random Number (0-1)() -> (number: 0 to 1=w457:dbl)
            }
            n111 = for {
              tunnel: w452 -> [w456] mode=indexing
              tunnel: [w455] -> w451 mode=indexing
              n112 = To Double Precision Float(number=w456) -> (double precision float=w455:dbl)
            }
            n113 = Build Array (concatenate)(w450, w451) -> (w449:dbl[])
          }
        }
        n114 = Initialize Array(0.0, w401) -> (w415:dbl[])
        n115 = RT FIFO Write(0:w408, 1:w407) -> (8:w405:refnum<k33>)  [unwired: 3 in, 3 out]
      }
    }
  }
  "error out" <- w2
